vi "期末專題_射飛機小遊戲.vi"() -> ()   [LabVIEW 2014]
panel:
  out "Game Over":picture
  out "Victory":picture
  in  "Total Score":dbl
  out "Airplane boom":picture
  out "Life":dbl(slide) scale=0.0..100.0
  out "Enemy Plane Boom":picture
  out "Enemy Plane \nNumber Left":dbl=10.0
  in  "Enemy Plane \nDown Speed":dbl(slide)=10.0 scale=10.0..30.0
  out "Enemy Plane":picture
  out "laser2":picture
  out "laser1":picture
  out "Airplane":picture
  out "Bckground":picture
  # "操作遊玩:\nStep1 : 藉由左邊拉桿可設定敵機降落速度\nStep2 : 敵機數量為10\nStep3 : 每擊落一架飛機得10分，分數超過60分即挑戰成功\nStep4 : 若不慎觸碰敵機則戰鬥機爆炸，結束遊戲Game over"
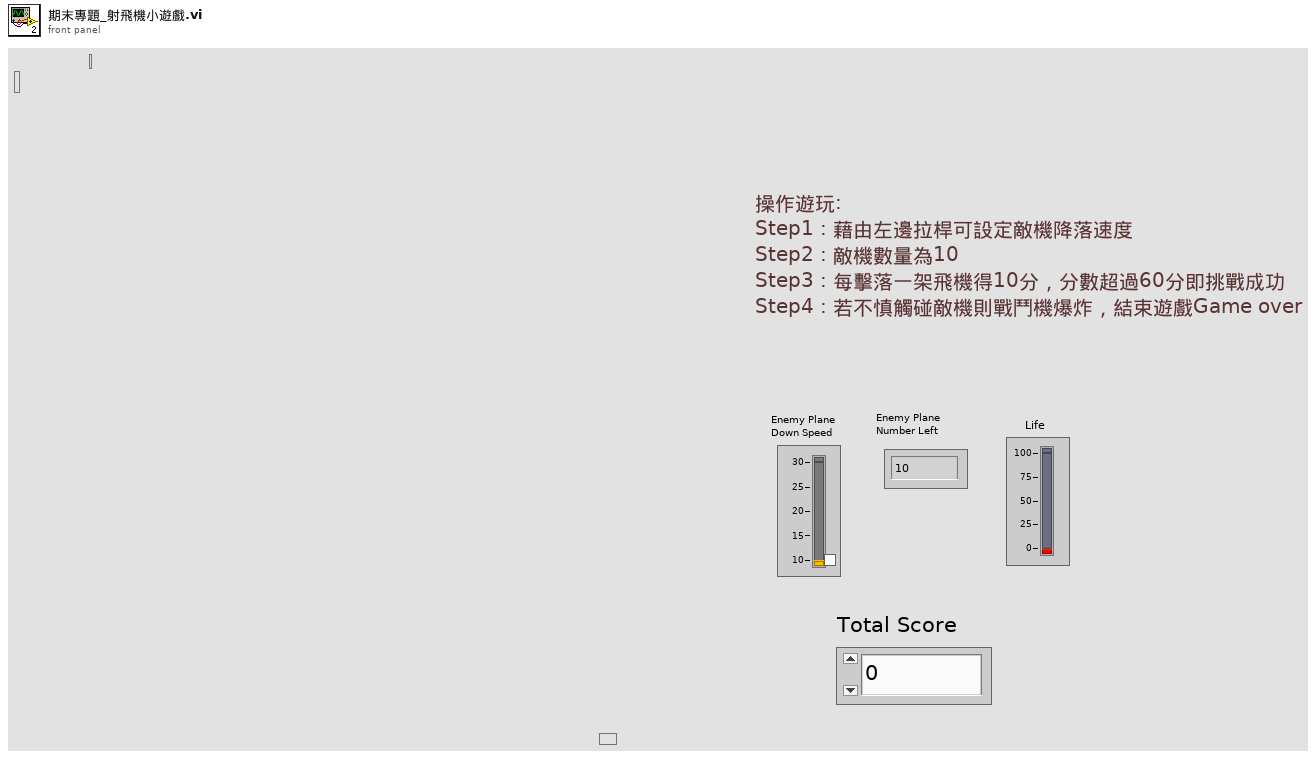
[diagram p1: front panel]
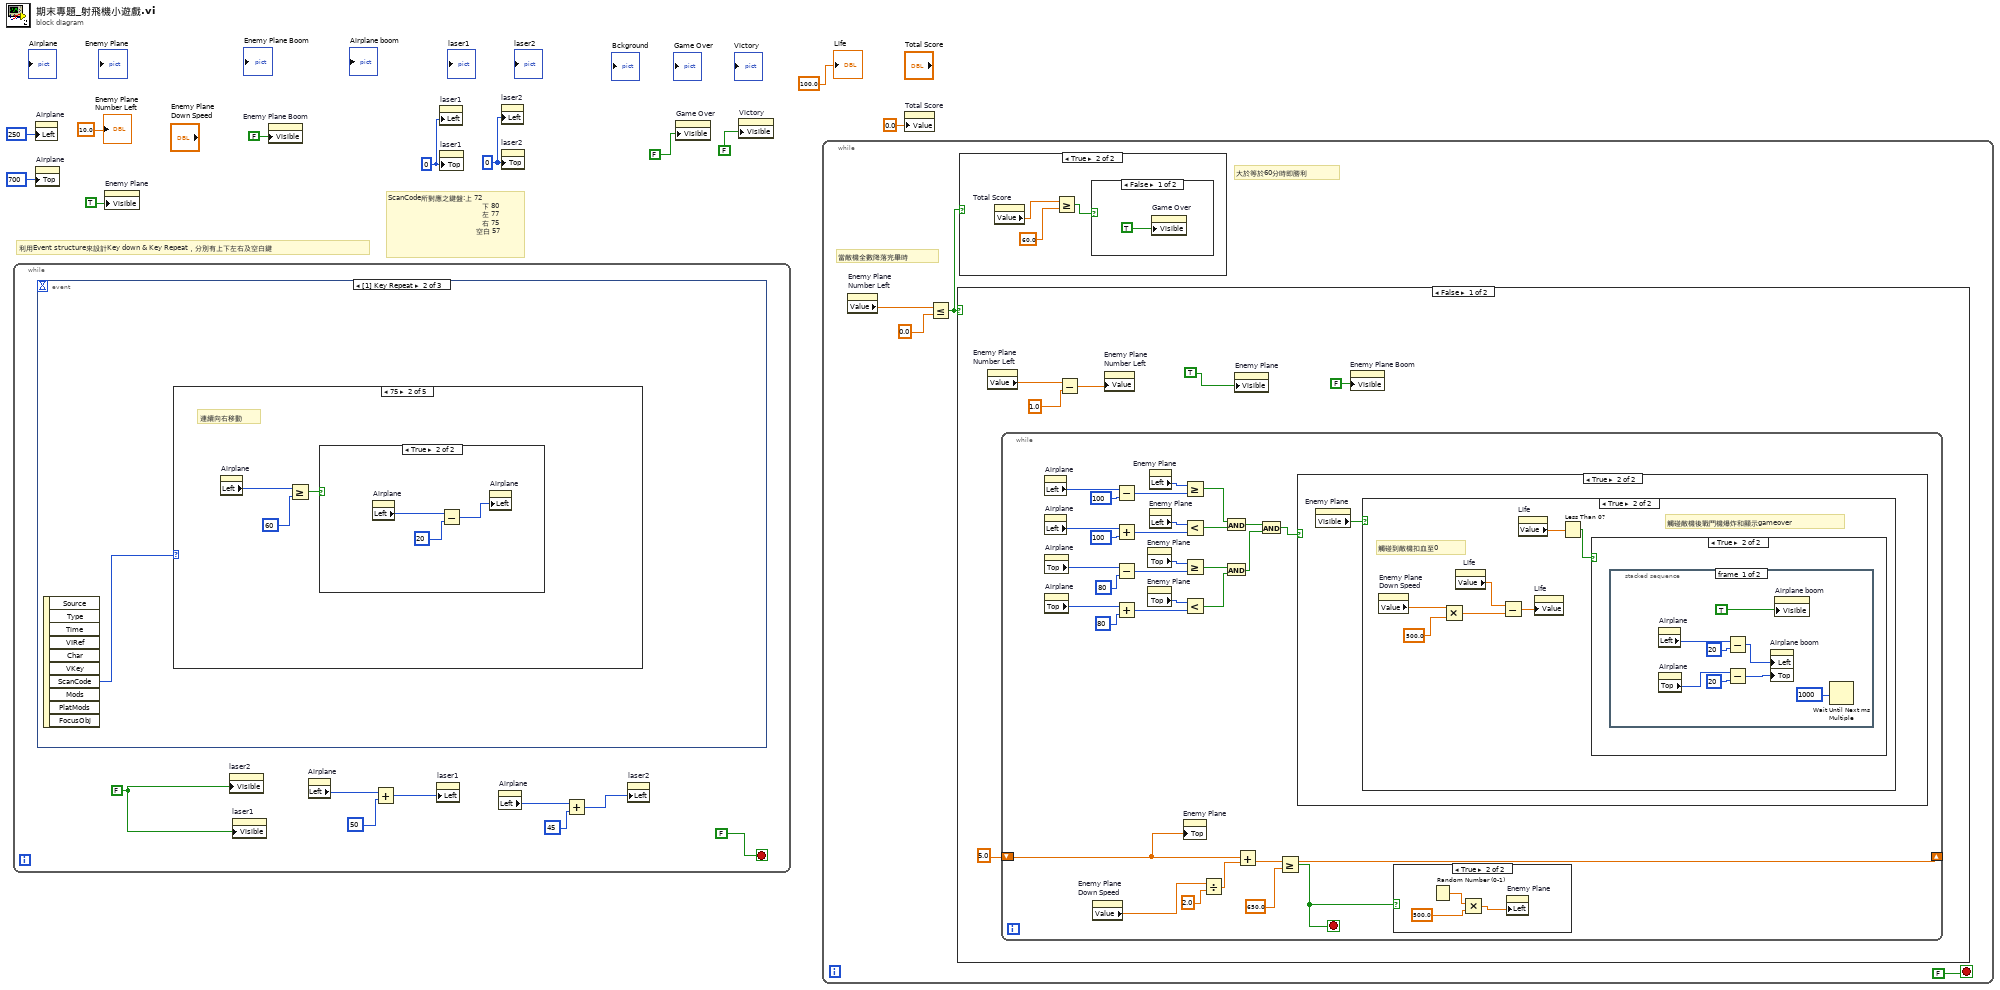
[diagram p0: block diagram]
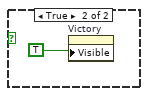
[diagram p3: hidden frame]
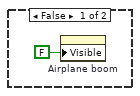
[diagram p5: hidden frame]
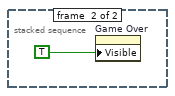
[diagram p8: hidden frame]
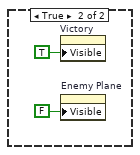
[diagram p9: hidden frame]
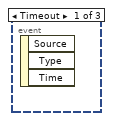
[diagram p10: hidden frame]
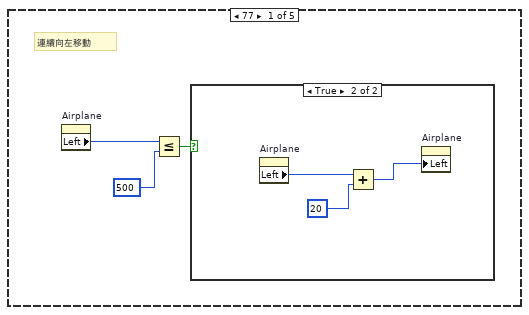
[diagram p11: hidden frame]
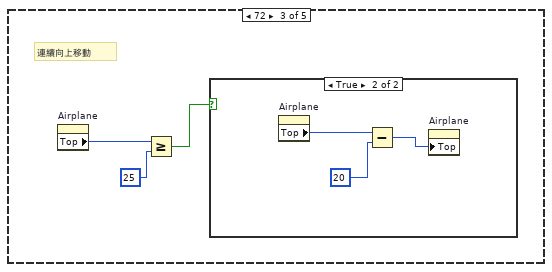
[diagram p14: hidden frame]
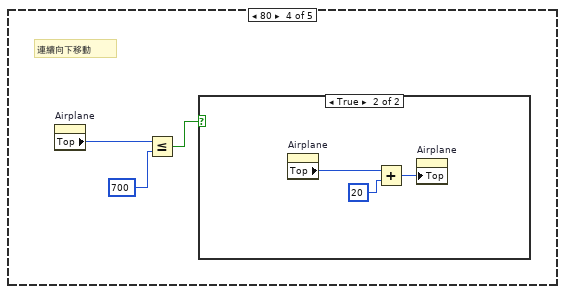
[diagram p16: hidden frame]
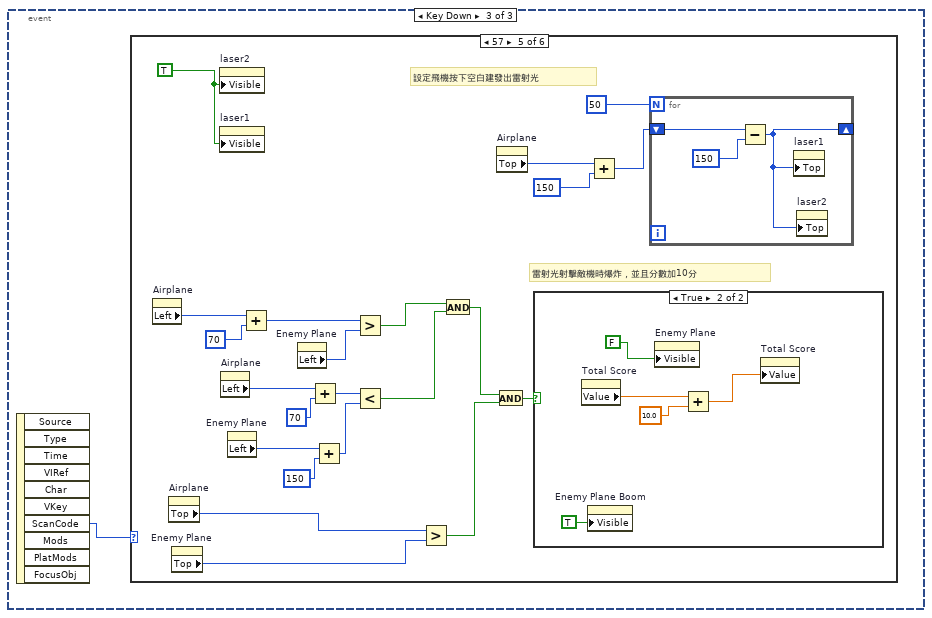
[diagram p19: hidden frame]
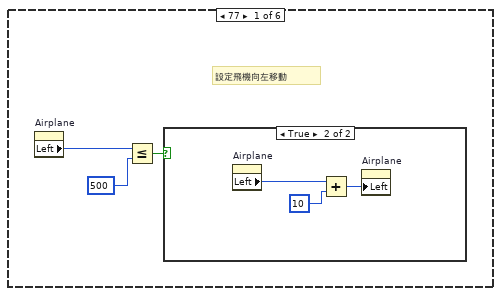
[diagram p20: hidden frame]
diagram:
  w8 = 0 ("Position:Top")
  w9 = 0 ("Position:Top")
  # "ScanCode所對應之鍵盤:上 72\n                                               下 80\n                                               左 77\n                                               右 75 \n                                            空白 57"
  # "利用Event structure來設計Key down & Key Repeat，分別有上下左右及空白鍵"
  n1 = while {
    stop <- FALSE stop-if-true
    w16 = FALSE
    n2 = event shown="[1] Key Repeat" {
      selector: _ -> [_ _ _]
      dyn-events: _ -> [_ _ _]
      timeout: _ -> [_ _ _]
      event Timeout {
        n3 = event-data() -> ()  [unwired: 1 in, 3 out]
      }
      event Key Repeat {
        n4 = event-data() -> ("ScanCode"=w20:i16)  [unwired: 1 in, 9 out]
        n5 = case shown="75" w20 {
          frame 77 {
            # "連續向左移動"
            n6 = property on="Airplane" class="Pict"() -> ("Left"=w23:i32)  [unwired: 2 in, 2 out]
            n7 = Less Or Equal?(x=w23, y=500) -> (x <= y?=w21:bool)
            n8 = case shown="True" w21 {
              frame False {
              }
              frame True {
                n9 = property on="Airplane" class="Pict"() -> ("Left"=w24:i32)  [unwired: 2 in, 2 out]
                n10 = Add(x=w24, y=20) -> (x+y=w26:i32)
                n11 = property on="Airplane" class="Pict"("Left"=w26) -> ()  [unwired: 2 in, 2 out]
              }
            }
          }
          frame 75 {
            # "連續向右移動"
            n12 = property on="Airplane" class="Pict"() -> ("Left"=w29:i32)  [unwired: 2 in, 2 out]
            n13 = Greater Or Equal?(x=w29, y=60) -> (x >= y?=w27:bool)
            n14 = case shown="True" w27 {
              frame False {
              }
              frame True {
                n15 = property on="Airplane" class="Pict"() -> ("Left"=w32:i32)  [unwired: 2 in, 2 out]
                n16 = Subtract(x=w32, y=20) -> (x-y=w30:i32)
                n17 = property on="Airplane" class="Pict"("Left"=w30) -> ()  [unwired: 2 in, 2 out]
              }
            }
          }
          frame 72 {
            # "連續向上移動"
            n18 = property on="Airplane" class="Pict"() -> ("Top"=w35:i32)  [unwired: 2 in, 2 out]
            n19 = Greater Or Equal?(x=w35, y=25) -> (x >= y?=w33:bool)
            n20 = case shown="True" w33 {
              frame False {
              }
              frame True {
                n21 = property on="Airplane" class="Pict"() -> ("Top"=w38:i32)  [unwired: 2 in, 2 out]
                n22 = Subtract(x=w38, y=20) -> (x-y=w36:i32)
                n23 = property on="Airplane" class="Pict"("Top"=w36) -> ()  [unwired: 2 in, 2 out]
              }
            }
          }
          frame 80 {
            # "連續向下移動"
            n24 = property on="Airplane" class="Pict"() -> ("Top"=w41:i32)  [unwired: 2 in, 2 out]
            n25 = Less Or Equal?(x=w41, y=700) -> (x <= y?=w39:bool)
            n26 = case shown="True" w39 {
              frame False {
              }
              frame True {
                n27 = property on="Airplane" class="Pict"() -> ("Top"=w44:i32)  [unwired: 2 in, 2 out]
                n28 = Add(x=w44, y=20) -> (x+y=w42:i32)
                n29 = property on="Airplane" class="Pict"("Top"=w42) -> ()  [unwired: 2 in, 2 out]
              }
            }
          }
          frame 0, Default {
          }
        }
      }
      event Key Down {
        n30 = event-data() -> ("ScanCode"=w45:i16)  [unwired: 1 in, 9 out]
        n31 = case shown="57" w45 {
          frame 77 {
            # "設定飛機向左移動"
            n32 = property on="Airplane" class="Pict"() -> ("Left"=w48:i32)  [unwired: 2 in, 2 out]
            n33 = Less Or Equal?(x=w48, y=500) -> (x <= y?=w46:bool)
            n34 = case shown="True" w46 {
              frame False {
              }
              frame True {
                n35 = property on="Airplane" class="Pict"() -> ("Left"=w49:i32)  [unwired: 2 in, 2 out]
                n36 = Add(x=w49, y=10) -> (x+y=w51:i32)
                n37 = property on="Airplane" class="Pict"("Left"=w51) -> ()  [unwired: 2 in, 2 out]
              }
            }
          }
          frame 75 {
            # "設定飛機向右移動"
            n38 = property on="Airplane" class="Pict"() -> ("Left"=w54:i32)  [unwired: 2 in, 2 out]
            n39 = Greater Or Equal?(x=w54, y=60) -> (x >= y?=w52:bool)
            n40 = case shown="True" w52 {
              frame False {
              }
              frame True {
                n41 = property on="Airplane" class="Pict"() -> ("Left"=w57:i32)  [unwired: 2 in, 2 out]
                n42 = Subtract(x=w57, y=10) -> (x-y=w55:i32)
                n43 = property on="Airplane" class="Pict"("Left"=w55) -> ()  [unwired: 2 in, 2 out]
              }
            }
          }
          frame 72 {
            # "設定飛機向上移動"
            n44 = property on="Airplane" class="Pict"() -> ("Top"=w60:i32)  [unwired: 2 in, 2 out]
            n45 = Greater Or Equal?(x=w60, y=25) -> (x >= y?=w58:bool)
            n46 = case shown="True" w58 {
              frame False {
              }
              frame True {
                n47 = property on="Airplane" class="Pict"() -> ("Top"=w63:i32)  [unwired: 2 in, 2 out]
                n48 = Subtract(x=w63, y=10) -> (x-y=w61:i32)
                n49 = property on="Airplane" class="Pict"("Top"=w61) -> ()  [unwired: 2 in, 2 out]
              }
            }
          }
          frame 80 {
            # "設定飛機向下移動"
            n50 = property on="Airplane" class="Pict"() -> ("Top"=w66:i32)  [unwired: 2 in, 2 out]
            n51 = Less Or Equal?(x=w66, y=700) -> (x <= y?=w64:bool)
            n52 = case shown="True" w64 {
              frame False {
              }
              frame True {
                n53 = property on="Airplane" class="Pict"() -> ("Top"=w69:i32)  [unwired: 2 in, 2 out]
                n54 = Add(x=w69, y=10) -> (x+y=w67:i32)
                n55 = property on="Airplane" class="Pict"("Top"=w67) -> ()  [unwired: 2 in, 2 out]
              }
            }
          }
          frame 57 {
            w89 = TRUE
            # "雷射光射擊敵機時爆炸，並且分數加10分"
            # "設定飛機按下空白建發出雷射光"
            n56 = property on="Airplane" class="Pict"() -> ("Left"=w72:i32)  [unwired: 2 in, 2 out]
            n57 = property on="Airplane" class="Pict"() -> ("Top"=w84:i32)  [unwired: 2 in, 2 out]
            n58 = property on="Enemy Plane" class="Pict"() -> ("Top"=w85:i32)  [unwired: 2 in, 2 out]
            n59 = property on="laser2" class="Pict"("Visible"=w89) -> ()  [unwired: 2 in, 2 out]
            n60 = property on="laser1" class="Pict"("Visible"=w89) -> ()  [unwired: 2 in, 2 out]
            n61 = property on="Airplane" class="Pict"() -> ("Left"=w78:i32)  [unwired: 2 in, 2 out]
            n62 = property on="Enemy Plane" class="Pict"() -> ("Left"=w79:i32)  [unwired: 2 in, 2 out]
            n63 = Add(x=w72, y=70) -> (x+y=w74:i32)
            n64 = property on="Enemy Plane" class="Pict"() -> ("Left"=w75:i32)  [unwired: 2 in, 2 out]
            n65 = Add(x=w78, y=70) -> (x+y=w76:i32)
            n66 = Add(x=w79, y=150) -> (x+y=w81:i32)
            n67 = Greater?(x=w74, y=w75) -> (0:w82:bool)
            n68 = Less?(x=w76, y=w81) -> (x < y?=w83:bool)
            n69 = Greater?(x=w84, y=w85) -> (0:w87:bool)
            n70 = And(x=w82, y=w83) -> (x .and. y?=w86:bool)
            n71 = And(x=w86, y=w87) -> (x .and. y?=w88:bool)
            n72 = property on="Airplane" class="Pict"() -> ("Top"=w91:i32)  [unwired: 2 in, 2 out]
            n73 = case shown="True" w88 {
              frame False {
              }
              frame True {
                n74 = property on="Total Score" class="DigNum (strict)"() -> ("Value"=w94:dbl)  [unwired: 2 in, 2 out]
                n75 = property on="Enemy Plane Boom" class="Pict"("Visible"=TRUE) -> ()  [unwired: 2 in, 2 out]
                n76 = property on="Enemy Plane" class="Pict"("Visible"=FALSE) -> ()  [unwired: 2 in, 2 out]
                n77 = Add(x=w94, y=10.0) -> (x+y=w95:dbl)
                n78 = property on="Total Score" class="DigNum (strict)"("Value"=w95) -> ()  [unwired: 2 in, 2 out]
              }
            }
            n79 = Add(x=w91, y=150) -> (x+y=w70:i32)
            n80 = for {
              N: 50 -> [_]
              shift-right: [w97] -> _
              shift-left: w70 -> [w99]
              n81 = Subtract(x=w99, y=150) -> (x-y=w97:i32)
              n82 = property on="laser1" class="Pict"("Top"=w97) -> ()  [unwired: 2 in, 2 out]
              n83 = property on="laser2" class="Pict"("Top"=w97) -> ()  [unwired: 2 in, 2 out]
            }
          }
          frame 0, Default {
          }
        }
      }
    }
    n84 = property on="laser2" class="Pict"("Visible"=w16) -> ()  [unwired: 2 in, 2 out]
    n85 = property on="laser1" class="Pict"("Visible"=w16) -> ()  [unwired: 2 in, 2 out]
    n86 = property on="Airplane" class="Pict"() -> ("Left"=w17:i32)  [unwired: 2 in, 2 out]
    n87 = Add(x=w17, y=50) -> (x+y=w19:i32)
    n88 = property on="laser1" class="Pict"("Left"=w19) -> ()  [unwired: 2 in, 2 out]
    n89 = property on="Airplane" class="Pict"() -> ("Left"=w12:i32)  [unwired: 2 in, 2 out]
    n90 = Add(x=w12, y=45) -> (x+y=w14:i32)
    n91 = property on="laser2" class="Pict"("Left"=w14) -> ()  [unwired: 2 in, 2 out]
  }
  n92 = property on="Airplane" class="Pict"("Left"=250 ("Position:Left")) -> ()  [unwired: 2 in, 2 out]
  n93 = property on="Airplane" class="Pict"("Top"=700 ("Position:Left")) -> ()  [unwired: 2 in, 2 out]
  n94 = property on="Enemy Plane" class="Pict"("Visible"=TRUE) -> ()  [unwired: 2 in, 2 out]
  n95 = property on="Enemy Plane Boom" class="Pict"("Visible"=FALSE) -> ()  [unwired: 2 in, 2 out]
  n96 = property on="laser1" class="Pict"("Left"=w8) -> ()  [unwired: 2 in, 2 out]
  n97 = property on="laser1" class="Pict"("Top"=w8) -> ()  [unwired: 2 in, 2 out]
  n98 = property on="laser2" class="Pict"("Left"=w9) -> ()  [unwired: 2 in, 2 out]
  n99 = property on="laser2" class="Pict"("Top"=w9) -> ()  [unwired: 2 in, 2 out]
  n100 = property on="Game Over" class="Pict"("Visible"=FALSE) -> ()  [unwired: 2 in, 2 out]
  n101 = property on="Victory" class="Pict"("Visible"=FALSE) -> ()  [unwired: 2 in, 2 out]
  n102 = while {
    stop <- FALSE stop-if-true
    # "大於等於60分時即勝利"
    # "當敵機全數降落完畢時"
    n103 = property on="Enemy Plane \nNumber Left" class="DigNum (strict)"() -> ("Value"=w103:dbl)  [unwired: 2 in, 2 out]
    n104 = Less Or Equal?(x=w103, y=0.0) -> (x <= y?=w100:bool)
    n105 = case shown="False" w100 {
      frame False {
        n106 = property on="Enemy Plane \nNumber Left" class="DigNum (strict)"() -> ("Value"=w111:dbl)  [unwired: 2 in, 2 out]
        n107 = while {
          shift-right: [w144] -> _
          shift-left: 5.0 -> [w116]
          stop <- w115 stop-if-true
          n108 = property on="Airplane" class="Pict"() -> ("Left"=w135:i32)  [unwired: 2 in, 2 out]
          n109 = property on="Airplane" class="Pict"() -> ("Left"=w133:i32)  [unwired: 2 in, 2 out]
          n110 = property on="Airplane" class="Pict"() -> ("Top"=w130:i32)  [unwired: 2 in, 2 out]
          n111 = property on="Airplane" class="Pict"() -> ("Top"=w126:i32)  [unwired: 2 in, 2 out]
          n112 = property on="Enemy Plane \nDown Speed" class="Slide (strict)"() -> ("Value"=w142:dbl)  [unwired: 2 in, 2 out]
          n113 = Subtract(x=w135, y=100) -> (x-y=w138:i32)
          n114 = Add(x=w133, y=100) -> (x+y=w137:i32)
          n115 = Subtract(x=w130, y=80) -> (x-y=w129:i32)
          n116 = Add(x=w126, y=80) -> (x+y=w125:i32)
          n117 = property on="Enemy Plane" class="Pict"() -> ("Top"=w131:i32)  [unwired: 2 in, 2 out]
          n118 = property on="Enemy Plane" class="Pict"() -> ("Top"=w127:i32)  [unwired: 2 in, 2 out]
          n119 = property on="Enemy Plane" class="Pict"() -> ("Left"=w134:i32)  [unwired: 2 in, 2 out]
          n120 = property on="Enemy Plane" class="Pict"() -> ("Left"=w132:i32)  [unwired: 2 in, 2 out]
          n121 = Greater Or Equal?(x=w134, y=w138) -> (x >= y?=w124:bool)
          n122 = Less?(x=w132, y=w137) -> (x < y?=w123:bool)
          n123 = Greater Or Equal?(x=w131, y=w129) -> (x >= y?=w122:bool)
          n124 = Less?(x=w127, y=w125) -> (x < y?=w121:bool)
          n125 = property on="Enemy Plane" class="Pict"("Top"=w116) -> ()  [unwired: 2 in, 2 out]
          n126 = Divide(x=w142, y=2.0) -> (x/y=w140:dbl)
          n127 = And(x=w124, y=w123) -> (x .and. y?=w119:bool)
          n128 = And(x=w122, y=w121) -> (x .and. y?=w120:bool)
          n129 = Add(x=w116, y=w140) -> (x+y=w144:dbl)
          n130 = And(x=w119, y=w120) -> (x .and. y?=w118:bool)
          n131 = Greater Or Equal?(x=w144, y=650.0) -> (x >= y?=w115:bool)
          n132 = case shown="True" w118 {
            frame False {
              n133 = property on="Airplane boom" class="Pict"("Visible"=FALSE) -> ()  [unwired: 2 in, 2 out]
            }
            frame True {
              n134 = property on="Enemy Plane" class="Pict"() -> ("Visible"=w149:bool)  [unwired: 2 in, 2 out]
              n135 = case shown="True" w149 {
                frame False {
                }
                frame True {
                  # "觸碰敵機後戰鬥機爆炸和顯示gameover"
                  # "觸碰到敵機扣血至0"
                  n136 = property on="Enemy Plane \nDown Speed" class="Slide (strict)"() -> ("Value"=w153:dbl)  [unwired: 2 in, 2 out]
                  n137 = Multiply(x=w153, y=500.0) -> (x*y=w150:dbl)
                  n138 = property on="Life" class="Slide (strict)"() -> ("Value"=w152:dbl)  [unwired: 2 in, 2 out]
                  n139 = Subtract(x=w152, y=w150) -> (x-y=w156:dbl)
                  n140 = property on="Life" class="Slide (strict)"() -> ("Value"=w155:dbl)  [unwired: 2 in, 2 out]
                  n141 = property on="Life" class="Slide (strict)"("Value"=w156) -> ()  [unwired: 2 in, 2 out]
                  n142 = Less Than 0?(x=w155) -> (x < 0?=w154:bool)
                  n143 = case shown="True" w154 {
                    frame False {
                    }
                    frame True {
                      n144 = stacked-sequence {
                        frame #0 {
                          n145 = property on="Airplane" class="Pict"() -> ("Left"=w159:i32)  [unwired: 2 in, 2 out]
                          n146 = property on="Airplane" class="Pict"() -> ("Top"=w162:i32)  [unwired: 2 in, 2 out]
                          n147 = Subtract(x=w159, y=20) -> (x-y=w160:i32)
                          n148 = Subtract(x=w162, y=20) -> (x-y=w164:i32)
                          n149 = property on="Airplane boom" class="Pict"("Left"=w160, "Top"=w164) -> ()  [unwired: 2 in, 2 out]
                          n150 = property on="Airplane boom" class="Pict"("Visible"=TRUE) -> ()  [unwired: 2 in, 2 out]
                          n151 = Wait Until Next ms Multiple(millisecond multiple=u32 1000) -> ()  [unwired: 1 out]
                        }
                        frame #1 {
                          n152 = property on="Game Over" class="Pict"("Visible"=TRUE) -> ()  [unwired: 2 in, 2 out]
                        }
                      }
                    }
                  }
                }
              }
            }
          }
          n153 = case shown="True" w115 {
            frame False {
            }
            frame True {
              n154 = Random Number (0-1)() -> (number: 0 to 1=w146:dbl)
              n155 = Multiply(x=w146, y=500.0) -> (x*y=w145:dbl)
              n156 = property on="Enemy Plane" class="Pict"("Left"=w145) -> ()  [unwired: 2 in, 2 out]
            }
          }
        }
        n157 = Subtract(x=w111, y=1.0) -> (x-y=w113:dbl)
        n158 = property on="Enemy Plane \nNumber Left" class="DigNum (strict)"("Value"=w113) -> ()  [unwired: 2 in, 2 out]
        n159 = property on="Enemy Plane" class="Pict"("Visible"=TRUE) -> ()  [unwired: 2 in, 2 out]
        n160 = property on="Enemy Plane Boom" class="Pict"("Visible"=FALSE) -> ()  [unwired: 2 in, 2 out]
      }
      frame True {
        n161 = property on="Victory" class="Pict"("Visible"=TRUE) -> ()  [unwired: 2 in, 2 out]
        n162 = property on="Enemy Plane" class="Pict"("Visible"=FALSE) -> ()  [unwired: 2 in, 2 out]
      }
    }
    n163 = case shown="True" w100 {
      frame False {
      }
      frame True {
        n164 = property on="Total Score" class="DigNum (strict)"() -> ("Value"=w106:dbl)  [unwired: 2 in, 2 out]
        n165 = Greater Or Equal?(x=w106, y=60.0) -> (x >= y?=w104:bool)
        n166 = case shown="False" w104 {
          frame False {
            n167 = property on="Game Over" class="Pict"("Visible"=TRUE) -> ()  [unwired: 2 in, 2 out]
          }
          frame True {
            n168 = property on="Victory" class="Pict"("Visible"=TRUE) -> ()  [unwired: 2 in, 2 out]
          }
        }
      }
    }
  }
  n169 = property on="Total Score" class="DigNum (strict)"("Value"=0.0 ("Score")) -> ()  [unwired: 2 in, 2 out]
  "Enemy Plane \nNumber Left" <- 10.0 ("Enemy Plane \n    Number")
  "Life" <- 100.0 ("Life")
